vi "Write State refnum from Value.vi"(8 "error in (no error)":errorcluster, 10 "States":T1, 11 "Generic Instrument.lvlib:Generic Card.lvclass":refnum<class "Generic Card.lvclass">) -> (0 "error out":errorcluster, 3 "Generic Card out":refnum<class "Generic Card.lvclass">)   [LabVIEW 2013, in "Generic Instrument.lvlib" / "Generic Card.lvclass"]
uses:
  Generic Card.lvclass
  Display Panel/Abstract Display/State.ctl
  Display Panel/Abstract Display/Abstract Display.lvclass
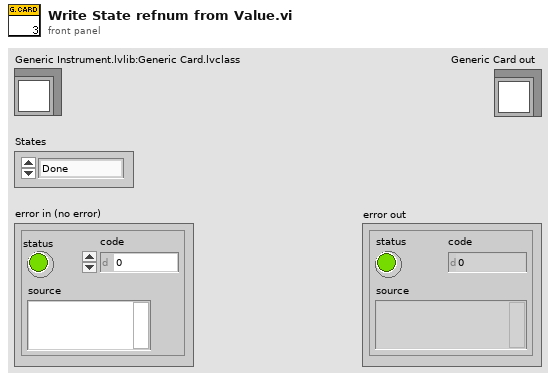
[diagram p1: front panel]
types:
  T1 = typedef "Display Panel.lvlib/Abstract Display.lvclass/State.ctl" = enum16{"Done", "Warming", "Measuring"}
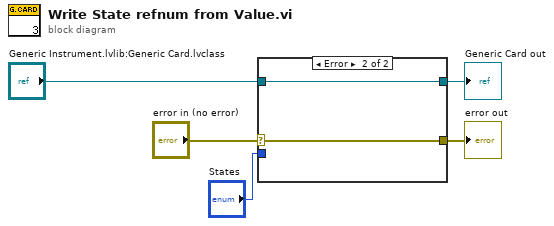
[diagram p0: block diagram]
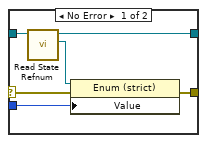
[diagram p2: hidden frame]
diagram:
  n1 = case shown="Error" "error in (no error)" {
    selector: "error in (no error)" -> [w8 w13]
    tunnel: "Generic Instrument.lvlib:Generic Card.lvclass" -> [w11 w12]
    tunnel: "States" -> [w9 _]
    tunnel: [w7 w12] -> w1
    tunnel: [w6 w13] -> w2
    frame No Error {
      n2 = call-dynamic "Read State Refnum.vi"("Generic Card in"=w11) -> ("State Refnum"=w10:refnum<vi>, "Generic Card out"=w7:refnum<class "Generic Card.lvclass">)  [unwired: 8 in, 1 out]
      n3 = property class="Enum (strict)"(reference=w10, error in=w8, "Value"=w9) -> (error out=w6:errorcluster)  [unwired: 1 out]
    }
    frame Error {
    }
  }
  "error out" <- w2
  "Generic Card out" <- w1
